vi "CRYSplit Comma String.vi"(10 "sSplit Letter":string=",", 11 "sData Out":string) -> (3 "Array":string[](array[string]))   [LabVIEW 2013]
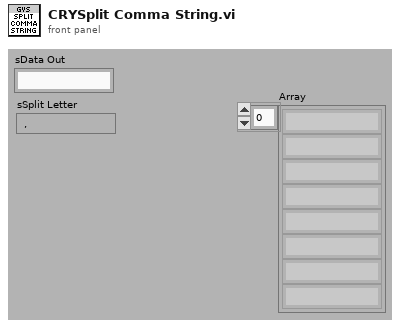
[diagram p1: front panel]
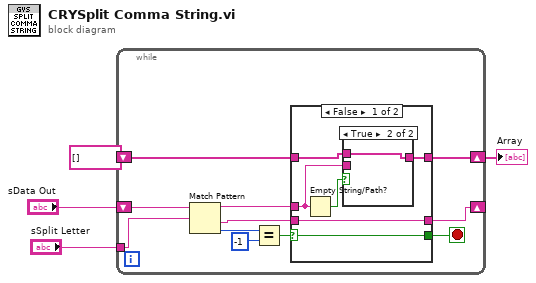
[diagram p0: block diagram]
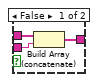
[diagram p2: hidden frame]
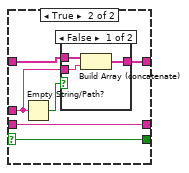
[diagram p3: hidden frame]
diagram:
  n1 = while {
    shift-right: [w9] -> w2
    shift-left: string[] [] ("Array") -> [w10]
    shift-right: [w6] -> _
    shift-left: "sData Out" -> [w15]
    tunnel: "sSplit Letter" -> [w5]
    stop <- w11 stop-if-true
    n2 = Match Pattern(string=w15, regular expression=w5) -> (before substring=w8:string, after substring=w7:string, offset past match=w14:i32)  [unwired: 1 in, 1 out]
    n3 = Equal?(x=w14, y=-1) -> (x = y?=w12:bool)
    n4 = case shown="False" w12 {
      selector: w12 -> [w21 w31]
      tunnel: [w21 w31] -> w11
      tunnel: [w18 w27] -> w9
      tunnel: w10 -> [w19 w29]
      tunnel: w8 -> [w17 w26]
      tunnel: [w20 w28] -> w6
      tunnel: w7 -> [w20 w28]
      frame False {
        n5 = Empty String/Path?(string/path=w17) -> (empty?=w16:bool)
        n6 = case shown="True" w16 {
          tunnel: w19 -> [w24 w25]
          tunnel: [w23 w25] -> w18
          tunnel: w17 -> [w22 _]
          frame False {
            n7 = Build Array (concatenate)(w24, w22) -> (w23:string[])
          }
          frame True {
          }
        }
      }
      frame True {
        n8 = Empty String/Path?(string/path=w26) -> (empty?=w30:bool)
        n9 = case shown="False" w30 {
          tunnel: w29 -> [w34 w35]
          tunnel: w26 -> [w33 _]
          tunnel: [w32 w35] -> w27
          frame False {
            n10 = Build Array (concatenate)(w34, w33) -> (w32:string[])
          }
          frame True {
          }
        }
      }
    }
  }
  "Array" <- w2
